vi "Ocean_Optics_Waveform.vi"() -> ()   [LabVIEW 2018]
doc: "Demonstrates continuous waveform measurement. Spectrum is displayed in a waveform graph."
uses:
  <instrlib>/Ocean Optics 2000 4000/Ocean Optics 2000 4000.lvlib
panel:
  in  "布尔":bool
  in  "文件路径":path
  out "半宽":dbl
  out "波长":dbl
  out "最大索引":i32
  out "峰值":dbl
  in  "Stop":bool
  out "Spectral Waveform":cluster{dbl[], dbl[]}(graph)
  in  "Enable Strobe (Disabled)":bool
  in  "VISA resource name":refnum<visa-resource-name>
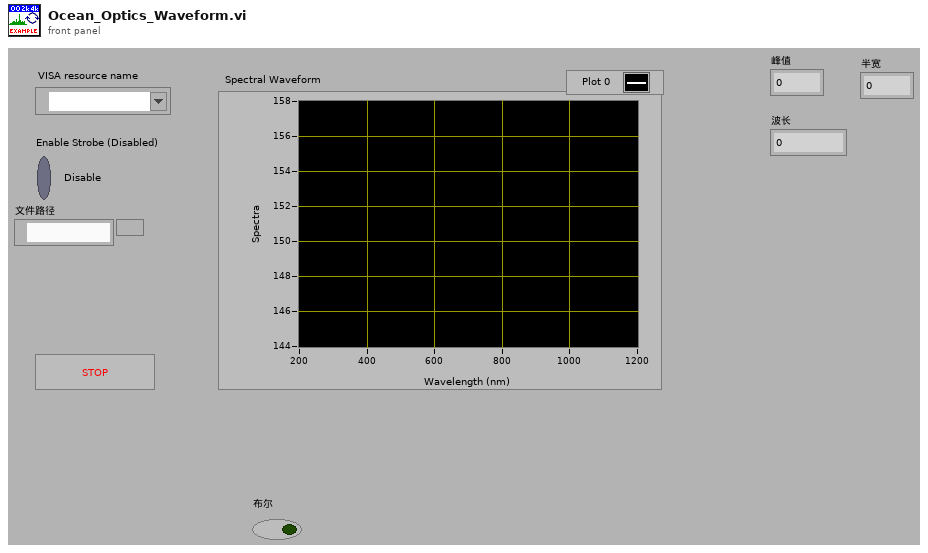
[diagram p1: front panel]
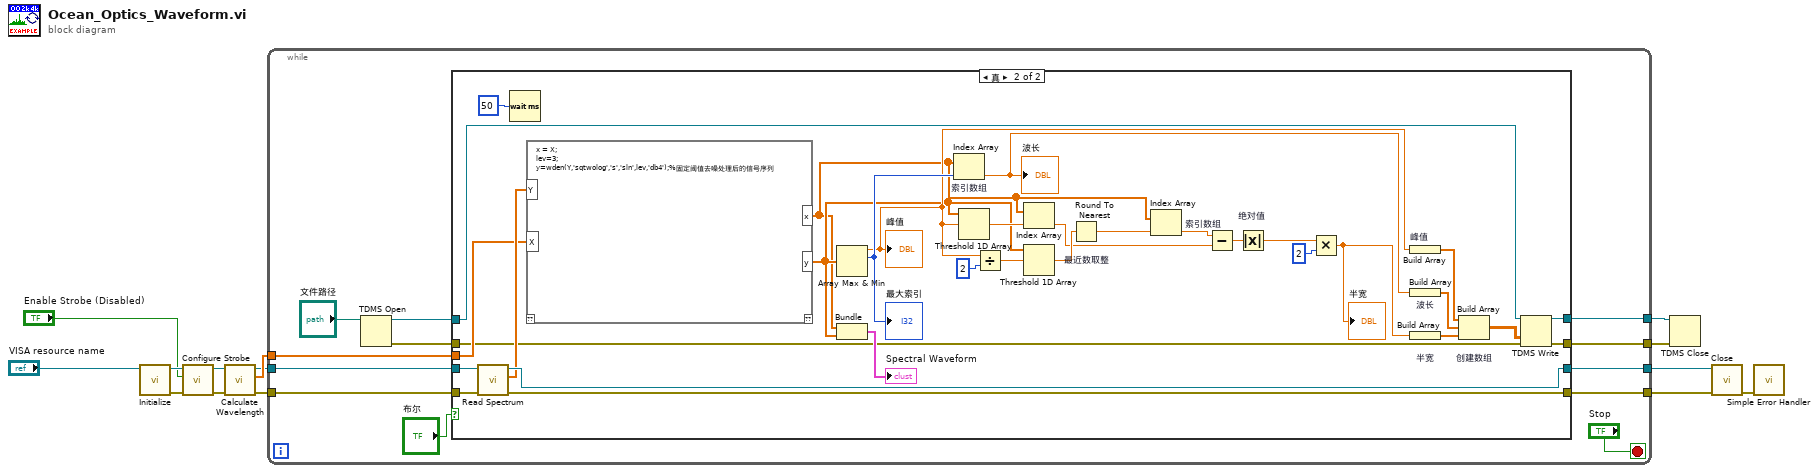
[diagram p0: block diagram]
diagram:
  n1 = call <instrlib>:"Initialize.vi"("VISA resource name"="VISA resource name") -> ("error out"=w13:errorcluster, "VISA resource name out"=w14:refnum<visa-resource-name>)  [unwired: 2 in, 7 out]
  n2 = call <instrlib>:"Configure Strobe.vi"("error in (no error)"=w13, "Enable Strobe (Disabled)"="Enable Strobe (Disabled)", "VISA resource name"=w14) -> ("error out"=w3:errorcluster, "VISA resource name out"=w4:refnum<visa-resource-name>)  [unwired: 7 out]
  n3 = call <instrlib>:"Calculate Wavelength.vi"("error in (no error)"=w3, "VISA resource name"=w4) -> ("error out"=w5:errorcluster, "Wavelength (nm)"=w7:dbl[], "VISA resource name out"=w6:refnum<visa-resource-name>)  [unwired: 1 in, 6 out]
  n4 = while {
    tunnel: [w20] -> w11
    tunnel: [w25] -> w10
    tunnel: w7 -> [w19]
    tunnel: w6 -> [w24]
    tunnel: w5 -> [w23]
    tunnel: [w22] -> w2
    tunnel: [w21] -> w1
    stop <- "Stop" stop-if-true
    n5 = TDMS Open(11:"文件路径") -> (0:w17:errorcluster, 3:w16:refnum<k34>)  [unwired: 6 in]
    n6 = case shown="真" "布尔" {
      tunnel: [_ w57] -> w25
      tunnel: w24 -> [_ w56]
      tunnel: w23 -> [_ w55]
      tunnel: [_ w43] -> w22
      tunnel: [_ w42] -> w21
      tunnel: [_ w34] -> w20
      tunnel: w19 -> [_ w31]
      tunnel: w17 -> [_ w28]
      tunnel: w16 -> [_ w27]
      frame False {
      }
      frame True {
        n7 = call <instrlib>:"Read Spectrum.vi"("error in (no error)"=w55, "VISA resource name"=w56) -> ("error out"=w57:errorcluster, "Spectrum by Pixel Number"=w32:dbl[], "VISA resource name out"=w34:refnum<visa-resource-name>)  [unwired: 6 in, 1 out]
        n8 = Wait (ms)(milliseconds to wait=u32 50 ("millisecond multiple")) -> ()  [unwired: 1 out]
        n9 = script code="x = X;\nlev=3;\ny=wden(Y,'sqtwolog','s','sln',lev,'db4');%固定阈值去噪处理后的信号序列"("Y"=w32, "X"=w31) -> ("x"=w29:dbl[], "y"=w30:dbl[])  [unwired: 1 in, 1 out]
        n10 = Array Max & Min(array=w30) -> (max value=w36:dbl, max index (indices)=w54:i32)  [unwired: 2 out]
        "峰值" <- w36
        "最大索引" <- w54
        n11 = Bundle(w29, w30) -> (→"Spectral Waveform":cluster{dbl[], dbl[]})  [unwired: 1 out]
        n12 = Index Array "索引数组"(array=w29, index=w54) -> (element=w37:dbl)
        "波长" <- w37
        n13 = Threshold 1D Array ("以阈值插值一维数组")(2:w36, 3:w30) -> (0:w49:dbl)  [unwired: 1 in]
        n14 = Divide(x=w36, y=2) -> (x/y=w50:dbl)
        n15 = Index Array(array=w29, index=w49) -> (element=w48:dbl)
        n16 = Threshold 1D Array(2:w50, 3:w30) -> (0:w52:dbl)  [unwired: 1 in]
        n17 = Round To Nearest "最近数取整"(number=w52) -> (nearest integer value=w51:dbl)
        n18 = Index Array "索引数组"(array=w29, index=w51) -> (element=w47:dbl)
        n19 = Subtract(x=w47, y=w48) -> (x-y=w46:dbl)
        n20 = Absolute Value "绝对值"(x=w46) -> (abs(x)=w45:dbl)
        n21 = Multiply(x=w45, y=2) -> (x*y=w39:dbl)
        "半宽" <- w39
        n22 = Build Array "峰值"(w36) -> (w35:dbl[])
        n23 = Build Array "波长"(w37) -> (w38:dbl[])
        n24 = Build Array "半宽"(w39) -> (w40:dbl[])
        n25 = Build Array "创建数组"(w35, w38, w40) -> (w41:dbl[][])
        n26 = TDMS Write(0:w27, 9:w41, 11:w28) -> (4:w43:refnum<k34>, 15:w42:errorcluster)  [unwired: 3 in, 2 out]
      }
    }
  }
  n27 = TDMS Close(8:w1, 11:w2) -> ()  [unwired: 2 out]
  n28 = call <instrlib>:"Close.vi"("error in (no error)"=w10, "VISA resource name"=w11) -> ("error out"=w9:errorcluster)  [unwired: 9 out]
  n29 = call <vilib>:"Simple Error Handler.vi"("error in (no error)"=w9) -> ()  [unwired: 1 in, 8 out]
